vi "PixelLineToGantryLine.vi"(8 "error in":errorcluster, 10 "cluster":T1 {"Start X" scale=0.0..1024.0; "End X" scale=0.0..1024.0}, 11 "Controller In":refnum<k24>) -> (0 "error out":errorcluster, 1 "intercept":dbl, 2 "slope":dbl, 3 "controller out":refnum<k24>, 4 "Angle(degree)":dbl)   [LabVIEW 2019]
uses:
  C:/Users/TTUHEP/Documents/LabVIEW/Other Models/2010/Bin/Aerotech.A3200.dll
  Other Models/2010/Bin/Aerotech.A3200.dll
  <vilib>/Analysis/NI_AALPro.lvlib
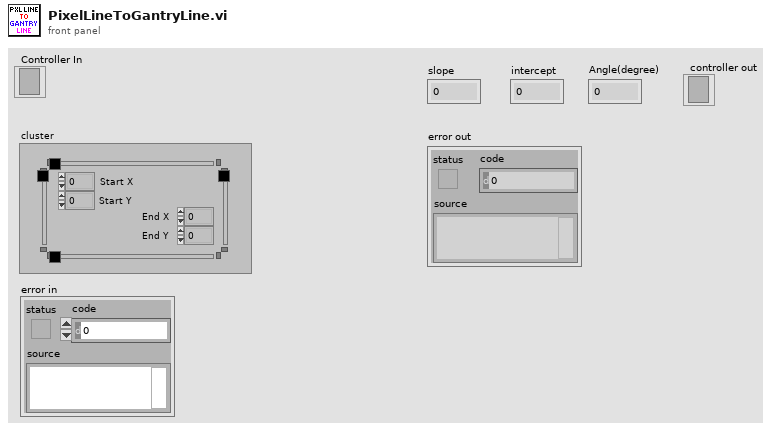
[diagram p1: front panel]
types:
  T1 = typedef "IMAQ Line" = cluster{"Start X":i32, "Start Y":i32, "End X":i32, "End Y":i32}
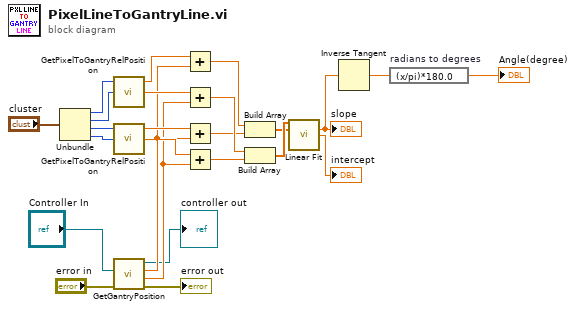
[diagram p0: block diagram]
diagram:
  n1 = Unbundle("cluster") -> ("Start X"=w22:i32, "Start Y"=w23:i32, "End X"=w24:i32, "End Y"=w25:i32)
  n2 = call "GetPixelToGantryRelPosition.vi"("PixelY"=w23, "PixelX"=w22) -> ("YmmRelGH"=w19:dbl, "XmmRelGH"=w16:dbl)  [unwired: 1 in, 1 out]
  n3 = call "GetPixelToGantryRelPosition.vi"("PixelY"=w25, "PixelX"=w24) -> ("YmmRelGH"=w20:dbl, "XmmRelGH"=w21:dbl)  [unwired: 1 in, 1 out]
  n4 = call "GetGantryPosition.vi"("error in (no error)"="error in", "Controller In"="Controller In") -> ("error out"=→"error out":errorcluster, "Position Y"=w6:dbl, "Position X"=w7:dbl, "controller out"=→"controller out":refnum<k24>)  [unwired: 3 in, 3 out]
  n5 = Add(x=w16, y=w7) -> (x+y=w15:dbl)
  n6 = Add(x=w19, y=w6) -> (x+y=w14:dbl)
  n7 = Add(x=w21, y=w7) -> (x+y=w13:dbl)
  n8 = Add(x=w20, y=w6) -> (x+y=w12:dbl)
  n9 = Build Array(w15, w13) -> (w17:dbl[])
  n10 = Build Array(w14, w12) -> (w18:dbl[])
  n11 = call <vilib>:"Linear Fit.vi"("Y"=w18, "X"=w17) -> ("slope"=w9:dbl, "intercept"=→"intercept":dbl)  [unwired: 9 in, 3 out]
  "slope" <- w9
  n12 = Inverse Tangent(1:w9) -> (0:w10:dbl)
  n13 = expression code="(x/pi)*180.0" "radians to degrees"(w10) -> (→"Angle(degree)":dbl)
